vi "FGV_Number of larger windows open.vi"(8 "error in (no error)":errorcluster, 11 "Function":enum16{"Reset", "Add one", "Reduce one", "Read"}(ring)) -> (0 "error out":errorcluster, 3 "Number of Larger Image windows open":i8)   [LabVIEW 2020]
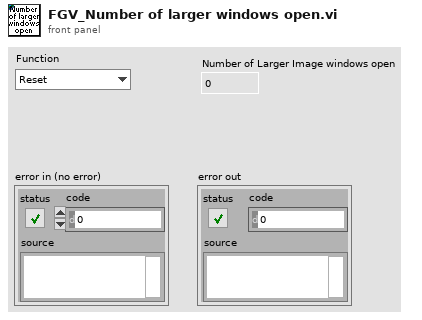
[diagram p1: front panel]
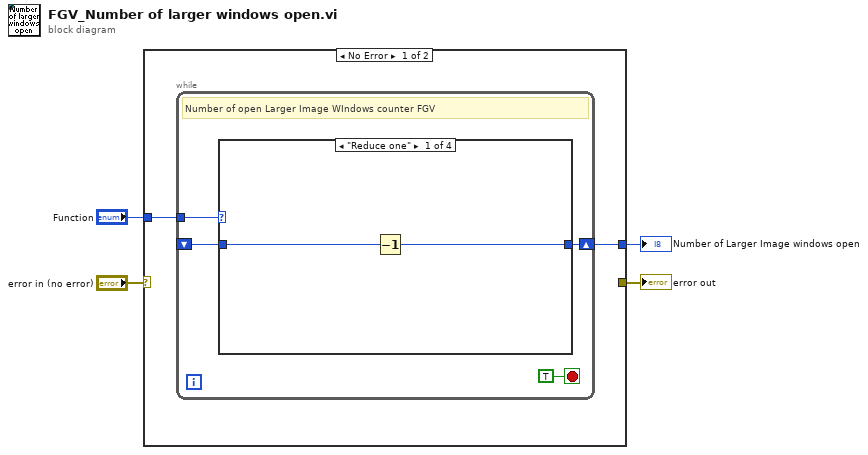
[diagram p0: block diagram]
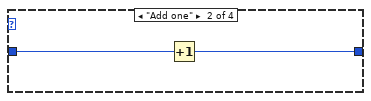
[diagram p2: hidden frame]
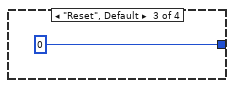
[diagram p3: hidden frame]
diagram:
  n1 = case shown="No Error" "error in (no error)" {
    selector: "error in (no error)" -> [_ w17]
    tunnel: [_ w17] -> w4
    tunnel: "Function" -> [w6 _]
    tunnel: [w5 _] -> w1
    frame No Error {
      n2 = while {
        shift-right: [w9] -> w5
        shift-left: _ -> [w8]
        tunnel: w6 -> [w7]
        stop <- TRUE stop-if-true
        # "Number of open Larger Image WIndows counter FGV"
        n3 = case shown="\"Reduce one\"" w7 {
          tunnel: [w11 w14 i8 0 w16] -> w9
          tunnel: w8 -> [w12 w13 _ w16]
          frame "Reduce one" {
            n4 = Decrement(x=w12) -> (x-1=w11:i8)
          }
          frame "Add one" {
            n5 = Increment(x=w13) -> (x+1=w14:i8)
          }
          frame "Reset", Default {
          }
          frame "Read" {
          }
        }
      }
    }
    frame Error {
    }
  }
  "error out" <- w4
  "Number of Larger Image windows open" <- w1
